vi "数采仪日志报警存储(子VI).vi"   [LabVIEW 2016, in "数据传输系统-03.lvlib"]
types:
  T1 = cluster{"时间标识":timestamp, "设备":string, "日志信息":string, "流程参数":string}
  T2 = typedef "报警信息字段定义.ctl" = cluster{"时间":timestamp, "参数":string, "报警信息":string, "备注":string, "code":u64}
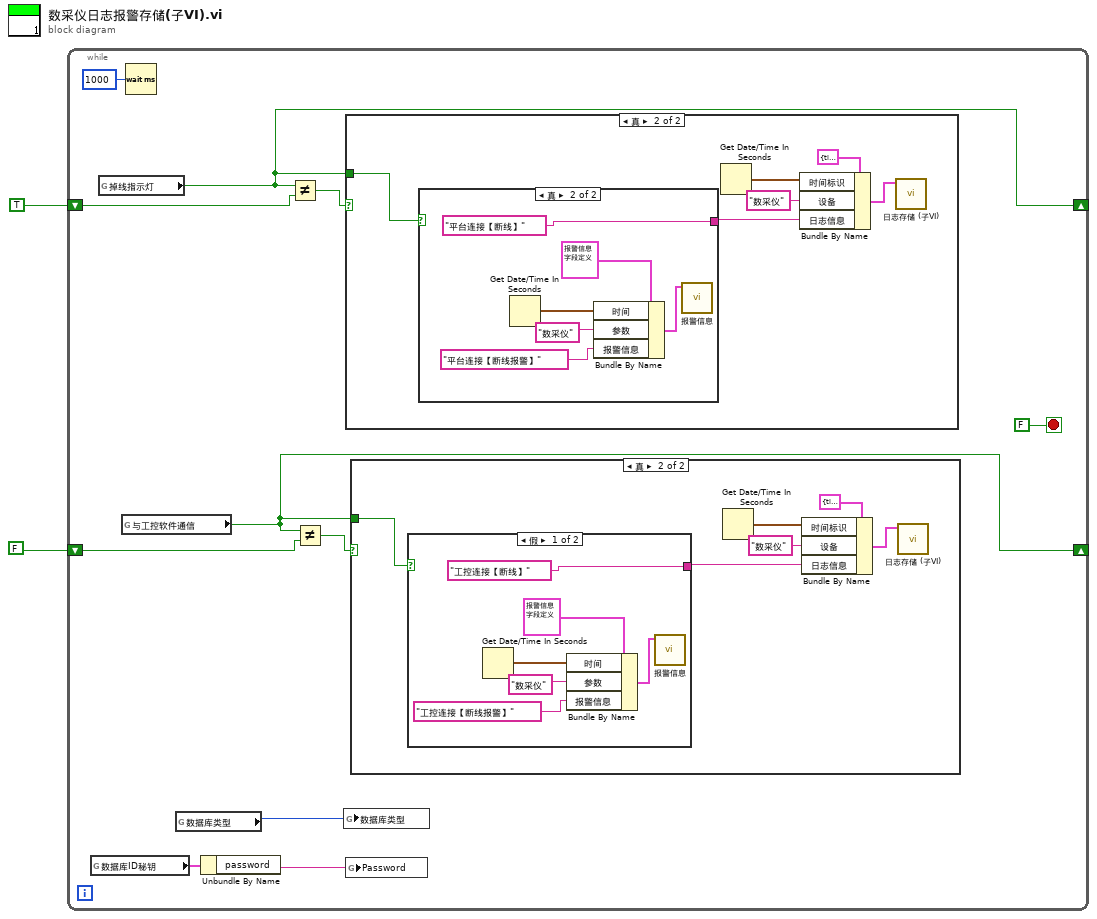
[diagram p0: block diagram]
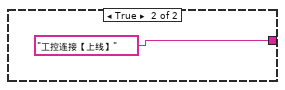
[diagram p3: hidden frame]
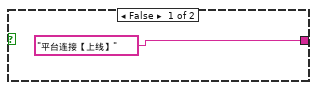
[diagram p5: hidden frame]
diagram:
  n1 = while {
    shift-right: [w9] -> _
    shift-left: TRUE -> [w10]
    shift-right: [w6] -> _
    shift-left: FALSE -> [w7]
    stop <- FALSE stop-if-true
    n2 = global read "外部交互全局.vi" "数据库ID秘钥"() -> (w5:cluster{"userID":string, "password":string})
    n3 = global read "全局 数据发送重叠.vi" "掉线指示灯"() -> (w9:bool)
    n4 = global read "全局1.vi" "与工控软件通信"() -> (w6:bool)
    n5 = Wait (ms)(milliseconds to wait=u32 1000 ("等待时间（毫秒）")) -> ()  [unwired: 1 out]
    n6 = global read "断电保存全局.vi" "数据库类型"() -> (w3:enum16{"Access", "SQLite"})
    n7 = Unbundle By Name(w5) -> ("password"=w4:string)
    n8 = Not Equal?(x=w9, y=w10) -> (x != y?=w11:bool)
    n9 = Not Equal?(x=w6, y=w7) -> (x != y?=w8:bool)
    n10 = global write "外部调用接口全局变量.vi" "数据库类型"(w3) -> ()
    n11 = case shown="真" w11 {
      tunnel: w9 -> [_ w27]
      frame False {
      }
      frame True {
        n12 = case shown="真" w27 {
          tunnel: ["平台连接【上线】" ("设备") "平台连接【断线】" ("设备")] -> w28
          frame False {
          }
          frame True {
            n13 = Get Date/Time In Seconds() -> (seconds since 1Jan1904=w38:timestamp)
            n14 = Bundle By Name(cluster=T2 {"时间"=timestamp(0 s since 1904-01-01), "参数"="", "报警信息"="", "备注"="", "code"=0} ("data"), "时间"=w38, "参数"="数采仪" ("设备"), "报警信息"="平台连接【断线报警】" ("设备")) -> (w34:T2)
            n15 = call "报警信息.vi"("data"=w34) -> ()  [unwired: 10 in, 1 out]
          }
        }
        n16 = Get Date/Time In Seconds() -> (seconds since 1Jan1904=w30:timestamp)
        n17 = Bundle By Name(cluster=T1 {"时间标识"=timestamp(0 s since 1904-01-01), "设备"="", "日志信息"="", "流程参数"=""} ("data in"), "时间标识"=w30, "设备"="数采仪", "日志信息"=w28) -> (w31:T1)
        n18 = call "日志存储 (子VI).vi"("data in"=w31) -> ()  [unwired: 11 in]
      }
    }
    n19 = global write "外部调用接口全局变量.vi" "Password"(w4) -> ()
    n20 = case shown="真" w8 {
      tunnel: w6 -> [_ w14]
      frame False {
      }
      frame True {
        n21 = case shown="假" w14 {
          tunnel: ["工控连接【断线】" ("设备") "工控连接【上线】" ("设备")] -> w15
          frame False {
            n22 = Get Date/Time In Seconds() -> (seconds since 1Jan1904=w23:timestamp)
            n23 = Bundle By Name(cluster=T2 {"时间"=timestamp(0 s since 1904-01-01), "参数"="", "报警信息"="", "备注"="", "code"=0} ("data"), "时间"=w23, "参数"="数采仪" ("设备"), "报警信息"="工控连接【断线报警】" ("设备")) -> (w24:T2)
            n24 = call "报警信息.vi"("data"=w24) -> ()  [unwired: 10 in, 1 out]
          }
          frame True {
          }
        }
        n25 = Get Date/Time In Seconds() -> (seconds since 1Jan1904=w17:timestamp)
        n26 = Bundle By Name(cluster=T1 {"时间标识"=timestamp(0 s since 1904-01-01), "设备"="", "日志信息"="", "流程参数"=""} ("data in"), "时间标识"=w17, "设备"="数采仪", "日志信息"=w15) -> (w18:T1)
        n27 = call "日志存储 (子VI).vi"("data in"=w18) -> ()  [unwired: 11 in]
      }
    }
  }
